vi "ConfigTasks.vi"(11 "Cluster In":T1[](array[typedef])) -> (2 "PXIs":refnum<k21>[](array[refnum]), 3 "PXI_Cluster":T1[](array[typedef]))   [LabVIEW 2013]
uses:
  AcqControls/Tasks_Indices.ctl
  Globals/Meas_global.vi
  <vilib>/DAQmx/configure/trigger.llb/DAQmx Start Trigger (Digital Edge).vi
  <vilib>/DAQmx/configure/timing.llb/DAQmx Timing (Sample Clock).vi
  <resource>/objmgr/daqmx.rc
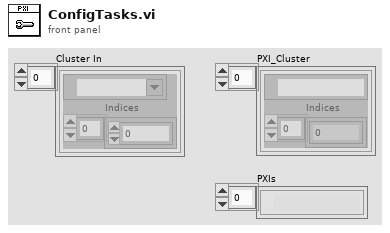
[diagram p1: front panel]
types:
  T1 = typedef "Tasks_Indices.ctl" = cluster{"task out":refnum<k21>, "Indices":i32[]}
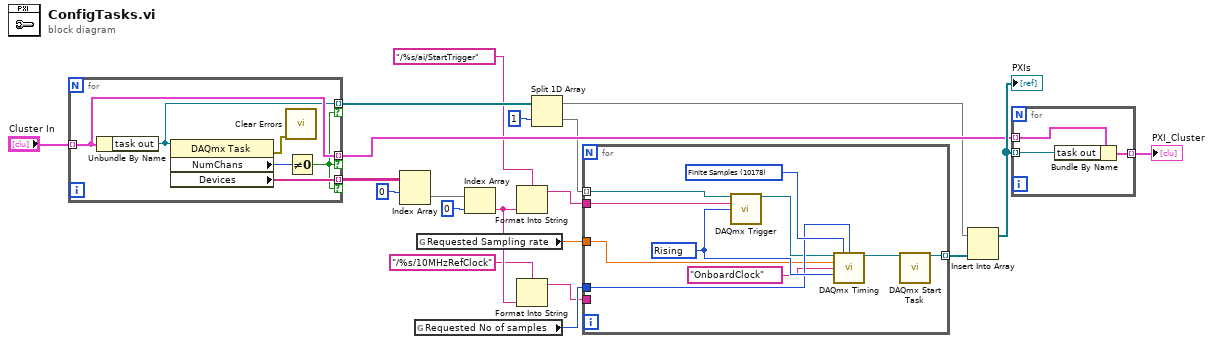
[diagram p0: block diagram]
diagram:
  n1 = for {
    tunnel: [w24] -> w18 mode=indexing if=w21
    tunnel: "Cluster In" -> [w24] mode=indexing
    tunnel: [w23] -> w8 mode=indexing if=w21
    tunnel: [w22] -> w3 mode=indexing if=w21
    n2 = Unbundle By Name(w24) -> ("task out"=w23:refnum<k21>)
    n3 = property class="DAQmx Task"(reference=w23) -> (error out=w25:errorcluster, "NumChans"=w26:u32, "Devices"=w22:tag[])  [unwired: 1 in, 1 out]
    n4 = call <vilib>:"Clear Errors.vi"("error in (no error)"=w25) -> ()  [unwired: 6 in, 1 out]
    n5 = Not Equal To 0?(x=w26) -> (x != 0?=w21:bool)
  }
  n6 = Index Array(array=w3, index (row)=0) -> (element=w5:tag[])  [unwired: 1 in]
  n7 = global read "Meas_global.vi" "Requested No of samples"() -> (w16:i32)
  n8 = global read "Meas_global.vi" "Requested Sampling rate"() -> (w17:dbl)
  n9 = Index Array(array=w5, index=0) -> (element=w14:tag)
  n10 = Format Into String(format string="/%s/ai/StartTrigger", w14) -> (resulting string=w10:string)  [unwired: 2 in, 1 out]
  n11 = Format Into String(format string="/%s/10MHzRefClock", w14) -> (resulting string=w15:string)  [unwired: 2 in, 1 out]
  n12 = Split 1D Array(array=w8, index=1) -> (first subarray=w11:refnum<k21>[], second subarray=w9:refnum<k21>[])
  n13 = for {
    tunnel: w9 -> [w36] mode=indexing
    tunnel: w10 -> [w35]
    tunnel: [w34] -> w12 mode=indexing
    tunnel: w15 -> [_]
    tunnel: w16 -> [w31]
    tunnel: w17 -> [w28]
    w33 = 10178 items=["Finite Samples"=10178, "Continuous Samples"=10123, "Hardware Timed Single Point"=12522] ("sample mode")
    w32 = 10280 items=["Rising"=10280, "Falling"=10171] ("edge")
    n14 = call-poly <vilib>:"DAQmx Trigger.vi"("task/channels in"=w36, "source"=w35, "edge"=w32) -> ("task out"=w29:refnum<k21>)  [unwired: 11 in, 1 out]
    n15 = call-poly <vilib>:"DAQmx Timing.vi"("task/channels in"=w29, "sample mode"=w33, "samples per channel"=w31, "rate"=w28, "source"=tag "OnboardClock", "active edge"=w32) -> ("task out"=w30:refnum<k21>)  [unwired: 8 in, 1 out]
    n16 = call <vilib>:"DAQmx Start Task.vi"("task/channels in"=w30) -> ("task out"=w34:refnum<k21>)  [unwired: 13 in, 1 out]
  }
  n17 = Insert Into Array(array=w11, new element=w12) -> (w20:refnum<k21>[])  [unwired: 1 in]
  "PXIs" <- w20
  n18 = for {
    tunnel: w20 -> [w38] mode=indexing
    tunnel: w18 -> [w39] mode=indexing
    tunnel: [w37] -> w19 mode=indexing
    n19 = Bundle By Name(cluster=w39, "task out"=w38) -> (w37:T1)
  }
  "PXI_Cluster" <- w19
